vi "Simple_LV2.vi"(0 "Data_In":dbl format="%#_13g", 11 "Error_In":errorcluster, 12 "Operation":T1 items=["Write", "Read"]) -> (4 "Data_Out":dbl format="%#_13g", 15 "Error_Out":errorcluster)   [LabVIEW 2023]
doc: "This a simply LV2 which can be write and read accross VIs"
uses:
  Type_Def/Operation_Simple_LV2.ctl
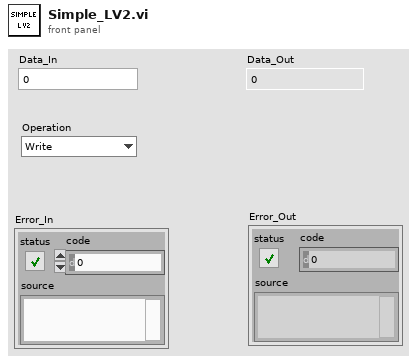
[diagram p1: front panel]
types:
  T1 = typedef "Operation_Simple_LV2.ctl" = u16
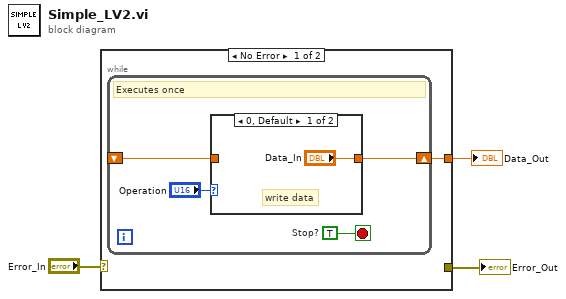
[diagram p0: block diagram]
diagram:
  n1 = case shown="No Error" "Error_In" {
    selector: "Error_In" -> [_ w11]
    tunnel: [_ w11] -> w2
    tunnel: [w4 _] -> w1
    frame No Error {
      n2 = while {
        shift-right: [w6] -> w4
        shift-left: _ -> [w5]
        stop <- w8 stop-if-true
        w8 = TRUE  # Stop?
        # "Executes once"
        n3 = case shown="0, Default" "Operation" {
          tunnel: ["Data_In" w10] -> w6
          tunnel: w5 -> [_ w10]
          frame 0, Default {
            # "write data"
          }
          frame 1 {
            # "Read data"
          }
        }
      }
    }
    frame Error {
    }
  }
  "Error_Out" <- w2
  "Data_Out" <- w1
